vi "ColorWheelDoppler.vi"(9 "clip value low (cm/s)":dbl, 10 "clip value high (cm/s)":dbl, 11 "vector":csg[][](array[numeric])) -> (2 "image":picture)   [LabVIEW 2022 SP3]
uses:
  <vilib>/picture/picture.llb/Draw True-Color Pixmap.vi
  <vilib>/Analysis/NI_AALPro.lvlib
panel:
  out "Y=(X-offset)/scale":dbl[][](array[numeric])
  out "Array":dbl[][](array[numeric])
  out "Intensity Graph":sgl[][](graph)
  out "min value":sgl
  out "max value":sgl
  in  "Picture":picture
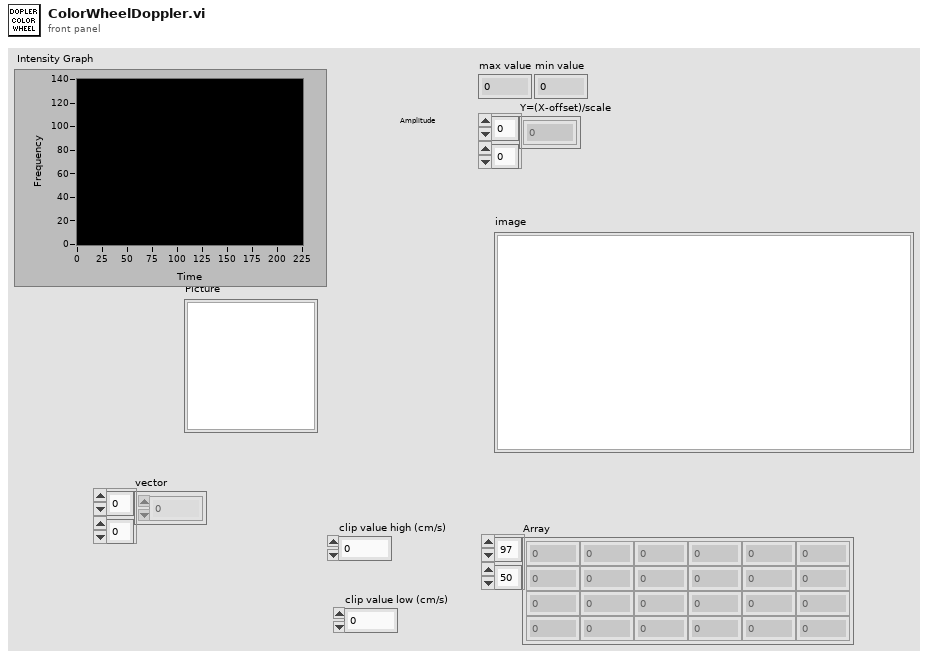
[diagram p1: front panel]
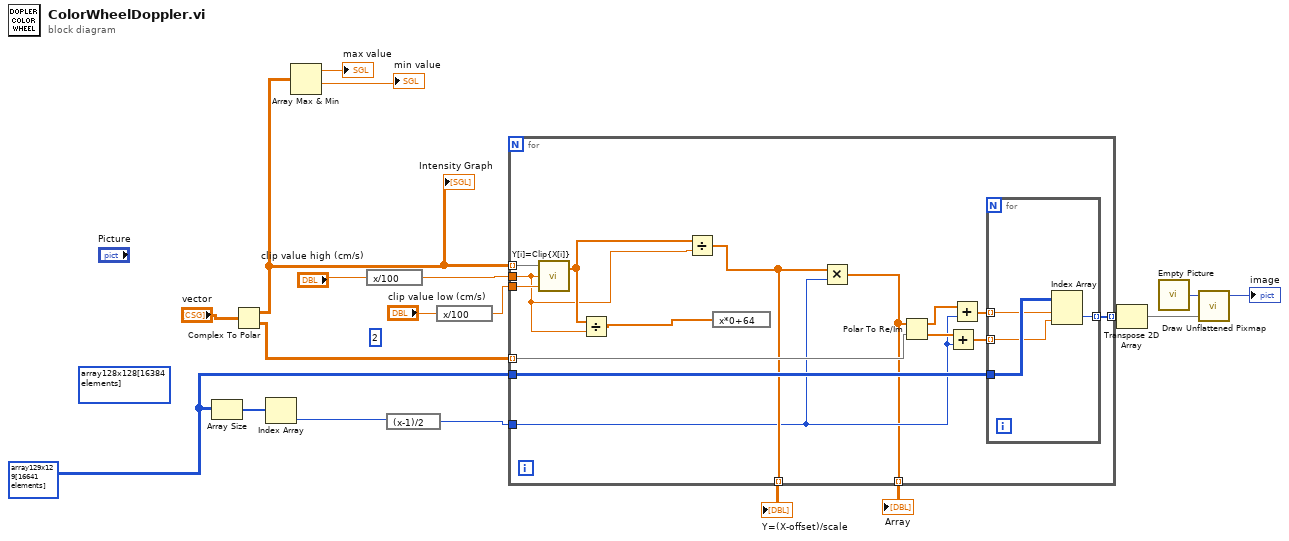
[diagram p0: block diagram]
diagram:
  w6 = u32[][] array129x129[16641 elements] ("True-color pixelmap")
  (unwired) 2
  (unwired) u32[][] array128x128[16384 elements] ("True-color pixelmap")
  n1 = Array Size(array=w6) -> (size(s)=w18:i32[])
  n2 = Complex To Polar(r * e^(i*theta)="vector") -> (r=w10:sgl[][], theta=w17:sgl[][])
  "Intensity Graph" <- w10
  n3 = Index Array(array=w18) -> (element=w5:i32)  [unwired: 1 in]
  n4 = Array Max & Min(array=w10) -> (max value=→"max value":sgl, min value=→"min value":sgl)  [unwired: 2 out]
  n5 = expression code="x/100"("clip value high (cm/s)") -> (w2:dbl)
  n6 = expression code="(x-1)/2"(w5) -> (w4:i32)
  n7 = expression code="x/100"("clip value low (cm/s)") -> (w1:dbl)
  n8 = for {
    tunnel: w10 -> [w27] mode=indexing
    tunnel: w17 -> [w34] mode=indexing
    tunnel: w4 -> [w21]
    tunnel: w6 -> [w31]
    tunnel: [w28] -> w14 mode=indexing
    tunnel: w1 -> [w26]
    tunnel: w2 -> [w23]
    tunnel: [w20] -> w7 mode=indexing
    tunnel: [w22] -> w3 mode=indexing
    n9 = call <vilib>:"Y[i]=Clip{X[i]}.vi"("lower limit"=w26, "upper limit"=w23, "Input Array"=w27) -> ("Clipped Array"=w24:dbl[])  [unwired: 1 out]
    n10 = Divide(x=w24, y=w23) -> (x/y=w25:dbl[])
    n11 = Divide(x=w24, y=w23) -> (x/y=w22:dbl[])
    n12 = expression code="x*0+64"(w25) -> ()  [unwired: 1 out]
    n13 = Multiply(x=w22, y=w21) -> (x*y=w20:dbl[])
    n14 = Polar To Re/Im(2:w34, 3:w20) -> (0:w33:dbl[], 1:w32:dbl[])
    n15 = Add(x=w33, y=w21) -> (x+y=w29:dbl[])
    n16 = Add(x=w32, y=w21) -> (x+y=w30:dbl[])
    n17 = for {
      tunnel: w31 -> [w38]
      tunnel: w30 -> [w37] mode=indexing
      tunnel: w29 -> [w36] mode=indexing
      tunnel: [w35] -> w28 mode=indexing
      n18 = Index Array(array=w38, index (row)=w37, index (col)=w36) -> (element=w35:u32)
    }
  }
  "Array" <- w7
  "Y=(X-offset)/scale" <- w3
  n19 = Transpose 2D Array(2D array=w14) -> (transposed array=w13:u32[][])
  n20 = call "Empty Picture"() -> ("empty picture"=w16:picture)
  n21 = call-poly <vilib>:"Draw Unflattened Pixmap.vi"("picture"=w16, "data (RGB format)"=w13) -> ("new picture"=→"image":picture)  [unwired: 7 in]
